vi "Cache-Move.vi"(6 "Time (now)":timestamp, 7 "Idx":i32, 8 "error in":errorcluster, 10 "Result in":T1) -> (0 "error out":errorcluster)   [LabVIEW 2016]
doc: "Go to DB->WriteStationValues action\nReturn boolean flag to show if data was saved to DB successfully\n\nWabco 2017 All right reserved\nAuthor: maciej.szupienko@wabco-auto.com"
uses:
  Cache.TestSteps.Fglb.ResultData.ctl
  Database/ProdaNG/Controls/ProdaNG.ProcessResult.ctl
  Database/ProdaNG/Controls/ProdaNG.ProcessStepResult.ctl
  Database/ProdaNG/Controls/ProdaNG.TestStepResult.ctl
  Database/ProdaNG/Controls/ProdaNG.TestValueResult.ctl
  Cache.Action.ctl
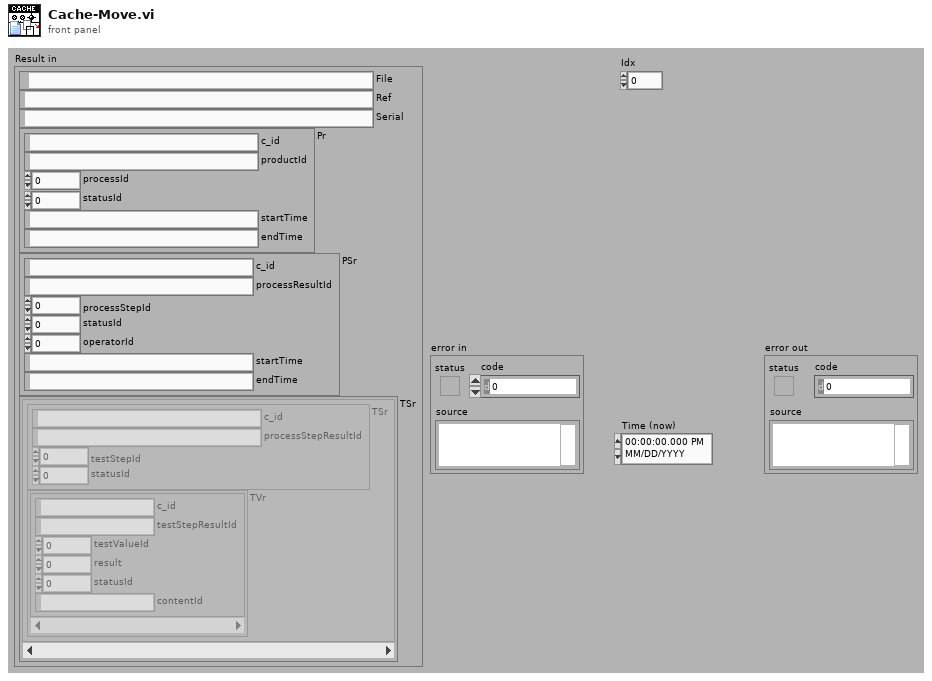
[diagram p1: front panel]
types:
  T1 = typedef "Cache.TestSteps.Fglb.ResultData.ctl" = cluster{"File":path, "Ref":string, "Serial":string, "Pr":T2, "PSr":T3, "TSr":cluster{"TSr":T4, "TVr":T5[]}[]}
  T2 = typedef "ProdaNG.ProcessResult.ctl" = cluster{"c_id":string, "productId":string, "processId":i32, "statusId":i32, "startTime":string, "endTime":string}
  T3 = typedef "ProdaNG.ProcessStepResult.ctl" = cluster{"c_id":string, "processResultId":string, "processStepId":i32, "statusId":i32, "operatorId":i32, "startTime":string, "endTime":string}
  T4 = typedef "ProdaNG.TestStepResult.ctl" = cluster{"c_id":string, "processStepResultId":string, "testStepId":i32, "statusId":i32}
  T5 = typedef "ProdaNG.TestValueResult.ctl" = cluster{"c_id":string, "testStepResultId":string, "testValueId":i32, "result":dbl, "statusId":i32, "contentId":string}
  T6 = typedef "Cache.Action.ctl" = enum32{"idle", "constructor", "destructor", "--- Cache ---", "Find", "FindToExport", "Move", "Delete"}
  T7 = cluster{"File":path, "Time (now)":timestamp, "error in":errorcluster}
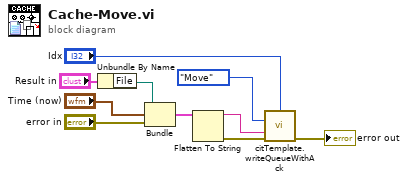
[diagram p0: block diagram]
diagram:
  n1 = Unbundle By Name("Result in") -> ("File"=w1:path)
  n2 = Bundle("File"=w1, "Time (now)"="Time (now)", "error in"="error in") -> (w5:T7)  [unwired: 1 in]
  n3 = Flatten To String(anything=w5) -> (data string=w9:string, error out=w8:errorcluster)  [unwired: 3 in, 1 out]
  n4 = call "citTemplate.writeQueueWithAck.vi"("instance (0)"="Idx", "event in"=Cache.Action."Move" ("Action"), "(flatten) data in"=w9, "error in (no error)"=w8) -> ("error out"=→"error out":errorcluster)  [unwired: 9 in, 2 out]
